vi "Test Suite Method Name Qualified.vi"(8 "error in (no error)":errorcluster, 11 "Test Case In":refnum<class "LUnit Test Suite Tests.lvclass">) -> (0 "error out":errorcluster, 3 "Test Case Out":refnum<class "LUnit Test Suite Tests.lvclass">)   [LabVIEW 2020, in "LUnit Test Suite Tests.lvclass"]
uses:
  LUnit Test Suite Tests.lvclass
  LUnit Test Suite Tests.lvclass/LUnit Test Suite Tests.ctl
  Mock Result Observer/Mock Result Observer.lvclass
  source/LUnit Test Suite.lvclass
  Test Doubles/Test Case Test Double/Test Case Test Double.lvclass
  <vilib>/Astemes/LUnit/Test Case.lvclass
  source/Framework/Single Thread Test Runner/Single Thread Test Runner.lvclass
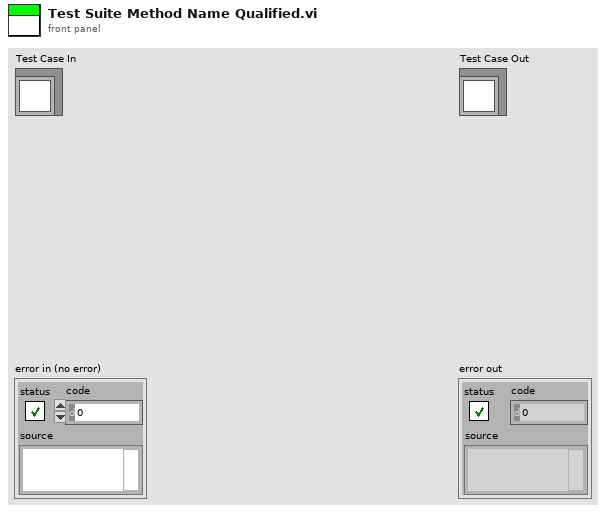
[diagram p1: front panel]
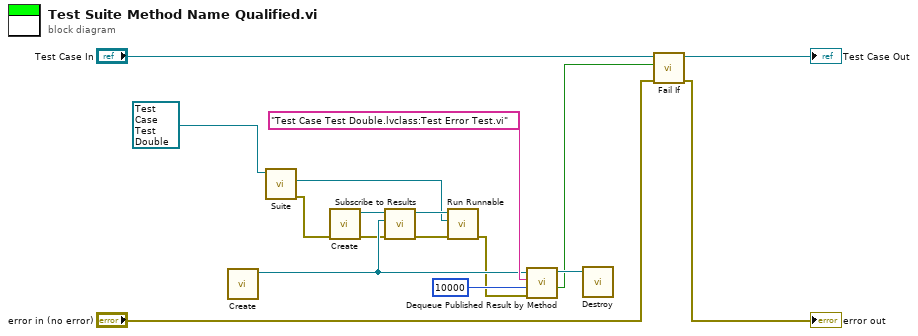
[diagram p0: block diagram]
diagram:
  n1 = call "Create.vi"() -> ("Mock Result Observer out"=w5:refnum<class "Mock Result Observer.lvclass">)  [unwired: 10 in, 1 out]
  n2 = call-dynamic "Suite.vi"("LUnit Test Case In"=refnum<class "Test Case Test Double.lvclass"> refnum ("LUnit Test Case V2 Test Double.lvclass")) -> ("error out"=w8:errorcluster, "LUnit Test Suite Out"=w2:refnum<class "LUnit Test Suite.lvclass">)  [unwired: 8 in, 1 out]
  n3 = call "Create.vi"("error in (no error)"=w8) -> ("error out"=w4:errorcluster, "Single Thread Test Runner out"=w3:refnum<class "Single Thread Test Runner.lvclass">)  [unwired: 9 in]
  n4 = call-dynamic "Subscribe to Results.vi"("error in (no error)"=w4, "Result Observer"=w5, "Single Thread Test Runner In"=w3) -> ("error out"=w6:errorcluster, "Single Thread Test Runner Out"=w7:refnum<class "Single Thread Test Runner.lvclass">)  [unwired: 7 in]
  n5 = call-dynamic "Run Runnable.vi"("error in (no error)"=w6, "Runnable"=w2, "Single Thread Test Runner In"=w7) -> ("error out"=w1:errorcluster)  [unwired: 7 in, 1 out]
  n6 = call "Dequeue Published Result by Method.vi"("error in (no error)"=w1, "timeout in ms"=10000, "Method Name"="Test Case Test Double.lvclass:Test Error Test.vi", "Mock Result Observer In"=w5) -> ("timed out?"=w9:bool, "Mock Result Observer Out"=w11:refnum<class "Mock Result Observer.lvclass">)  [unwired: 4 in, 2 out]
  n7 = call "Destroy.vi"("Mock Result Observer in"=w11) -> ()  [unwired: 9 in, 2 out]
  n8 = call <vilib>:"Fail If.vi"("error in (no error)"="error in (no error)", "Fail?"=w9, "LUnit Test Case In"="Test Case In") -> ("error out"=→"error out":errorcluster, "LUnit Test Case Out"=→"Test Case Out":refnum<class "LUnit Test Suite Tests.lvclass">)  [unwired: 7 in]
